vi "Write userEventFPGAVIRef.vi"(8 "error in (no error)":errorcluster, 10 "userEventFPGAVIRef":refnum<user-event>, 11 "CompactRIO in":refnum<class "CompactRIO.lvclass">) -> (0 "error out":errorcluster, 3 "CompactRIO out":refnum<class "CompactRIO.lvclass">)   [LabVIEW 2015, in "CompactRIO.lvclass"]
uses:
  CompactRIO.lvclass
  ComponentTemplateCore/ComponentModel/ComponentModelRT/Typedefs/FPGAVIRefCRIO9074.ctl
  CompactRIO.lvclass/CompactRIO.ctl
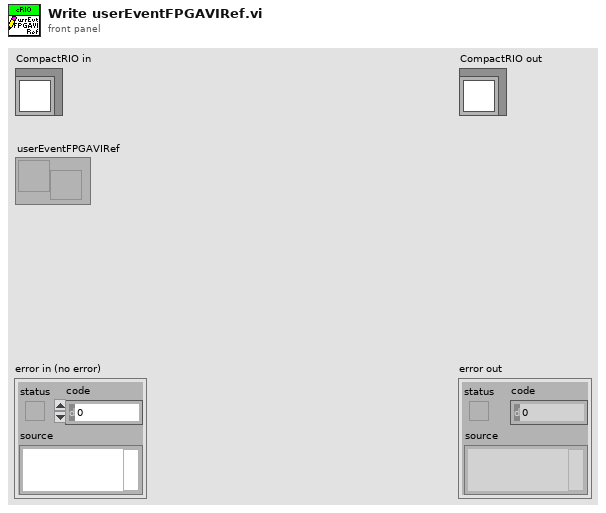
[diagram p1: front panel]
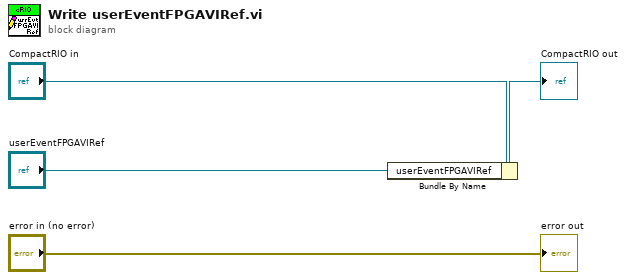
[diagram p0: block diagram]
diagram:
  n1 = Bundle By Name(cluster="CompactRIO in", "userEventFPGAVIRef"="userEventFPGAVIRef") -> (→"CompactRIO out":refnum<class "CompactRIO.lvclass">)
  "error out" <- "error in (no error)"
